vi "Read Joystick State.vi"(8 "error in (no error)":errorcluster, 11 "Comp XBox One Controller in":refnum<class "Comp XBox One Controller.lvclass">) -> (0 "error out":errorcluster, 2 "Joystick State":cluster{"Buttons":T1[], "Axis":T2[]}, 3 "Comp XBox One Controller out":refnum<class "Comp XBox One Controller.lvclass">)   [LabVIEW 2014, in "Comp XBox One Controller.lvlib" / "Comp XBox One Controller.lvclass"]
uses:
  Comp XBox One Controller.lvclass
  Robot/Joystick/Joystick Class/Button State.ctl
  Robot/Joystick/Joystick Class/Axis State.ctl
  Comp XBox One Controller.lvclass/Comp XBox One Controller.ctl
  Robot/Xbox One Controller/XBox One Controller Class/XBox One Controller.lvclass
  Robot/Joystick/Joystick Class/Joystick.lvclass
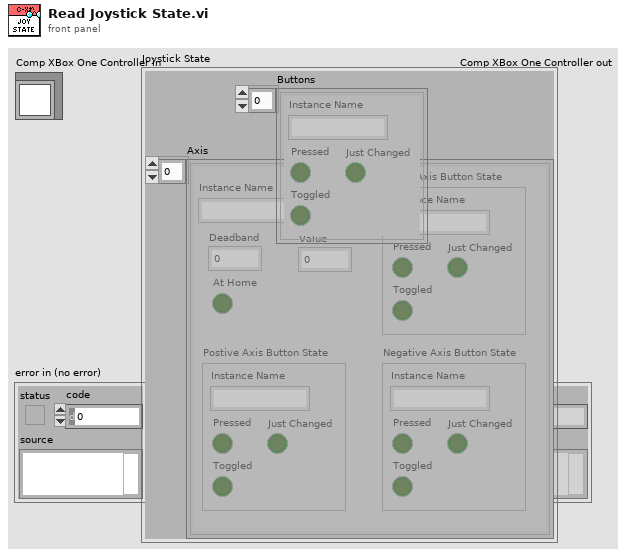
[diagram p1: front panel]
types:
  T1 = typedef "Joystick.lvlib/Joystick.lvclass/Button State.ctl" = cluster{"Pressed":bool, "Instance Name":string, "Toggled":bool, "Just Changed":bool}
  T2 = typedef "Joystick.lvlib/Joystick.lvclass/Axis State.ctl" = cluster{"Instance Name":string, "Deadband":dbl, "Value":dbl, "At Home":bool, "Postive Axis Button State":T1, "Negative Axis Button State":T1, "Home Axis Button State":T1}
  T3 = typedef "WPI_JoystickDevRef.ctl" = cluster{"Device":T4}
  T4 = typedef "WPI_JoystickDeviceEnum.ctl" = enum16{"USB 0", "USB 1", "USB 2", "USB 3", "USB 4", "USB 5"}
  T5 = typedef "Joystick.lvlib/Joystick.lvclass/Joystick State.ctl" = cluster{"Buttons":T1[], "Axis":T2[]}
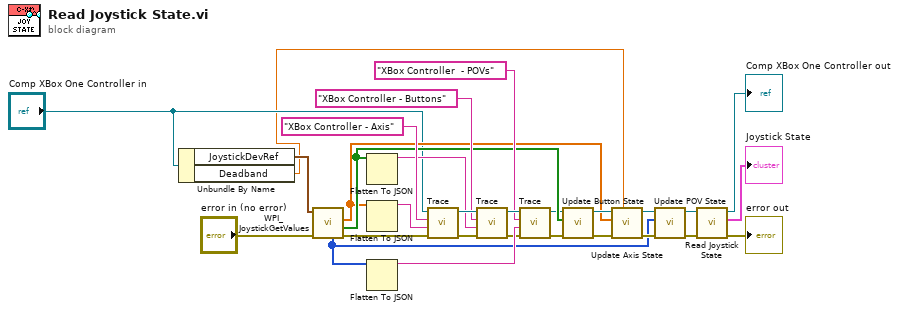
[diagram p0: block diagram]
diagram:
  n1 = Unbundle By Name("Comp XBox One Controller in") -> ("JoystickDevRef"=w29:T3, "Deadband"=w6:dbl)
  n2 = call <vilib>:"WPI_JoystickGetValues.vi"("error in (no error)"="error in (no error)", "JoystickDevRef"=w29) -> ("error out"=w11:errorcluster, "Buttons"=w19:bool[], "Axes"=w17:dbl[], "POVs"=w1:i16[])  [unwired: 5 in, 1 out]
  n3 = Flatten To JSON(anything=w19) -> (JSON string=w22:string)  [unwired: 2 in, 1 out]
  n4 = Flatten To JSON(anything=w17) -> (JSON string=w27:string)  [unwired: 2 in, 1 out]
  n5 = Flatten To JSON(anything=w1) -> (JSON string=w21:string)  [unwired: 2 in, 1 out]
  n6 = call-dynamic "Trace.vi"("error in (no error)"=w11, "System Message"=w27, "System Action"="XBox Controller - Axis", "System Actor in"="Comp XBox One Controller in") -> ("error out"=w20:errorcluster, "System Actor out"=w25:refnum<class "Comp XBox One Controller.lvclass">)  [unwired: 6 in]
  n7 = call-dynamic "Trace.vi"("error in (no error)"=w20, "System Message"=w22, "System Action"="XBox Controller - Buttons", "System Actor in"=w25) -> ("error out"=w14:errorcluster, "System Actor out"=w26:refnum<class "Comp XBox One Controller.lvclass">)  [unwired: 6 in]
  n8 = call-dynamic "Trace.vi"("error in (no error)"=w14, "System Message"=w21, "System Action"="XBox Controller  - POVs", "System Actor in"=w26) -> ("error out"=w10:errorcluster, "System Actor out"=w13:refnum<class "Comp XBox One Controller.lvclass">)  [unwired: 6 in]
  n9 = call-dynamic "Update Button State.vi"("error in (no error)"=w10, "Current Buttons"=w19, "Joystick in"=w13) -> ("error out"=w9:errorcluster, "Joystick out"=w18:refnum<class "Comp XBox One Controller.lvclass">)  [unwired: 7 in]
  n10 = call-dynamic "Update Axis State.vi"("Axis Deadband"=w6, "error in (no error)"=w9, "Axes"=w17, "Joystick in"=w18) -> ("error out"=w4:errorcluster, "Joystick out"=w5:refnum<class "Comp XBox One Controller.lvclass">)  [unwired: 6 in]
  n11 = call-dynamic "Update POV State.vi"("error in (no error)"=w4, "POVs"=w1, "Joystick in"=w5) -> ("error out"=w2:errorcluster, "Joystick out"=w3:refnum<class "Comp XBox One Controller.lvclass">)  [unwired: 7 in]
  n12 = call-parent "Read Joystick State.vi"("error in (no error)"=w2, "Joystick in"=w3) -> ("error out"=→"error out":errorcluster, "Joystick State"=→"Joystick State":T5, "Joystick out"=→"Comp XBox One Controller out":refnum<class "Comp XBox One Controller.lvclass">)  [unwired: 7 in]
